vi "PID Test.vi"() -> ()   [LabVIEW 2017]
uses:
  <vilib>/addons/control/pid/pid.llb/PID (DBL).vi
  <vilib>/addons/control/pid/NI_PID_pid.lvlib
panel:
  out "PID Output":dbl(graph)
  out "SP & PV":T1(graph)
  out "Velocity (mm/s)":dbl
  in  "PID gains":T2={"proportional gain (Kc)"=1.0, "integral time (Ti, min)"=0.01, "derivative time (Td, min)"=0.0} {"derivative time (Td, min)" format="%.3f"; "integral time (Ti, min)" format="%.3f"; "proportional gain (Kc)" format="%.3f"}
  out "dt out (s)":dbl format="%.3f"
  in  "FWD/RVS":bool
  in  "Frequency":dbl
  in  "Velocity Set Pt":dbl(slide) scale=0.0..30.0
  in  "stop":bool
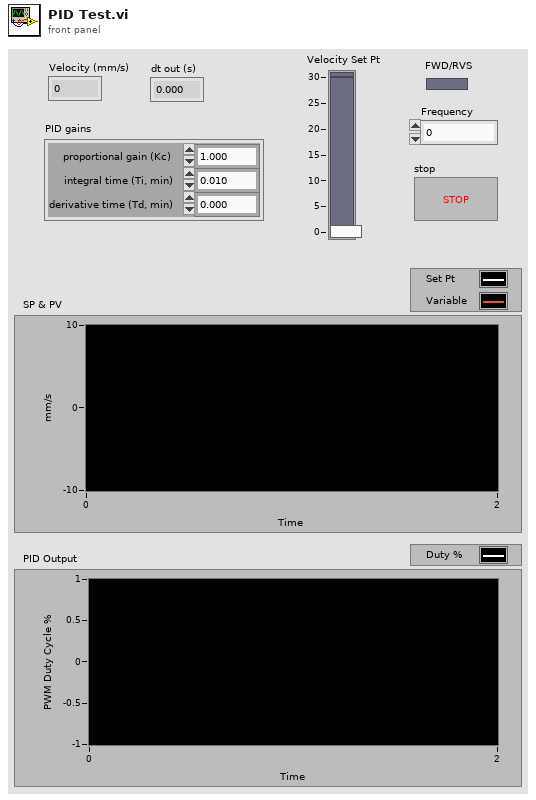
[diagram p1: front panel]
types:
  T1 = cluster{"Velocity Set Pt":dbl, "Velocity (mm/s)":dbl}
  T2 = cluster{"proportional gain (Kc)":dbl, "integral time (Ti, min)":dbl, "derivative time (Td, min)":dbl}
  T3 = typedef "Encoder Cluster.ctl" = cluster{"Y-axis rev count":dbl, "Y-axis distance":dbl, "X-axis rev count":dbl, "X-axis distance":dbl, "Y-axis direction":T4, "X-axis direction":T4, "X-counter val":i32, "Y-counter val":i32}
  T4 = typedef "Encoder Count Direction Enum.ctl" = enum16{"Counting Up", "Counting Down"}
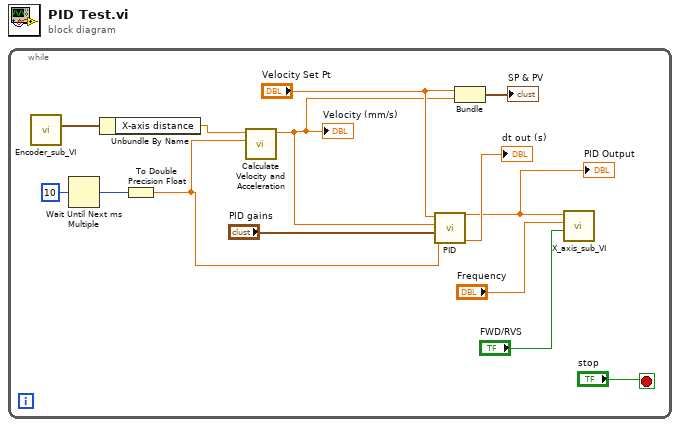
[diagram p0: block diagram]
diagram:
  n1 = while {
    stop <- "stop" stop-if-true
    n2 = call "Encoder_sub_VI.vi"() -> ("Encoder Output"=w11:T3)  [unwired: 10 in, 1 out]
    n3 = Wait Until Next ms Multiple(millisecond multiple=u32 10) -> (millisecond timer value=w8:u32)
    n4 = Unbundle By Name(w11) -> ("X-axis distance"=w10:dbl)
    n5 = To Double Precision Float(number=w8) -> (double precision float=w7:dbl)
    n6 = call "Calculate Velocity and Acceleration.vi"("Loop Runtime (s)"=w7, "Displacement (mm)"=w10) -> ("Velocity (mm/s)"=w2:dbl)  [unwired: 8 in, 1 out]
    "Velocity (mm/s)" <- w2
    n7 = call-poly <vilib>:"PID.vi"("dt (s)"=w7, "PID gains"="PID gains", "process variable"=w2, "setpoint"="Velocity Set Pt") -> ("dt out (s)"=→"dt out (s)":dbl, "output"=w1:dbl)  [unwired: 6 in]
    "PID Output" <- w1
    n8 = Bundle("Velocity Set Pt"="Velocity Set Pt", "Velocity (mm/s)"=w2) -> (→"SP & PV":T1)  [unwired: 1 in]
    n9 = call "X_axis_sub_VI.vi"("FWD/RVS"="FWD/RVS", "Frequency"="Frequency", "Duty Cycle %"=w1) -> ()  [unwired: 8 in, 1 out]
  }
